vi "HEWH RLT PRAT.vi"() -> ()   [LabVIEW 2023] (continued)
            n1006 = call <vilib>:"Add State(s) to Queue__jki_lib_state_machine.vi"("State(s) in (\"\")"=w2472) -> ("States Out"=w2471:string)  [unwired: 14 in]
          }
          frame "Test: Update Display C" {
            n1007 = local read "Appliance Details C"() -> (w2473:T5)
            n1008 = local read "Current (C)"() -> (w2482:dbl)
            n1009 = Bundle By Name(cluster=w2483, "Station C Display.Display Data (RLT).Current Display"=w2482, "Station C Display.Appliance Details"=w2473) -> (w2481:T97)
            n1010 = Unbundle By Name(w2481) -> ("Station C Display.Display Data (RLT).Station Label Display"=w2479:string, "Station C Display.Display Data (RLT).Board ID Display"=w2478:string, "Station C Display.Display Data (RLT).Serial Number Display"=w2477:string, "Station C Display.Display Data (RLT).Current Display"=w2476:dbl, "Station C Display.Display Data (RLT).Status Color"=w2475:u32, "Station C Display.Display Data (RLT).Cycle Count Display"=w2474:i32)
            n1011 = property on="Station Label Display" class="Str"("Value"=w2479) -> ()  [unwired: 2 in, 2 out]
            n1012 = property on="Board ID Display" class="Str"("Value"=w2478) -> ()  [unwired: 2 in, 2 out]
            n1013 = property on="Serial Number Display" class="Str"("Value"=w2477) -> ()  [unwired: 2 in, 2 out]
            n1014 = property on="Current Display" class="DigNum (strict)"("Value"=w2476) -> ()  [unwired: 2 in, 2 out]
            n1015 = property on="Status Color" class="ColBox"("Value"=w2475) -> ()  [unwired: 2 in, 2 out]
            n1016 = property on="Cycle Count Display" class="DigNum (strict)"("Value"=w2474) -> ()  [unwired: 2 in, 2 out]
            n1017 = call <vilib>:"Add State(s) to Queue__jki_lib_state_machine.vi"("State(s) in (\"\")"=w2486) -> ("States Out"=w2485:string)  [unwired: 14 in]
          }
          frame "Test: Update Display D" {
            n1018 = local read "Appliance Details D"() -> (w2487:T5)
            n1019 = local read "Current (D)"() -> (w2496:dbl)
            n1020 = Bundle By Name(cluster=w2497, "Station D Display.Display Data (RLT).Current Display"=w2496, "Station D Display.Appliance Details"=w2487) -> (w2495:T97)
            n1021 = Unbundle By Name(w2495) -> ("Station D Display.Display Data (RLT).Station Label Display"=w2493:string, "Station D Display.Display Data (RLT).Board ID Display"=w2492:string, "Station D Display.Display Data (RLT).Serial Number Display"=w2491:string, "Station D Display.Display Data (RLT).Current Display"=w2490:dbl, "Station D Display.Display Data (RLT).Status Color"=w2489:u32, "Station D Display.Display Data (RLT).Cycle Count Display"=w2488:i32)
            n1022 = property on="Station Label Display" class="Str"("Value"=w2493) -> ()  [unwired: 2 in, 2 out]
            n1023 = property on="Board ID Display" class="Str"("Value"=w2492) -> ()  [unwired: 2 in, 2 out]
            n1024 = property on="Serial Number Display" class="Str"("Value"=w2491) -> ()  [unwired: 2 in, 2 out]
            n1025 = property on="Current Display" class="DigNum (strict)"("Value"=w2490) -> ()  [unwired: 2 in, 2 out]
            n1026 = property on="Status Color" class="ColBox"("Value"=w2489) -> ()  [unwired: 2 in, 2 out]
            n1027 = property on="Cycle Count Display" class="DigNum (strict)"("Value"=w2488) -> ()  [unwired: 2 in, 2 out]
            n1028 = call <vilib>:"Add State(s) to Queue__jki_lib_state_machine.vi"("State(s) in (\"\")"=w2500) -> ("States Out"=w2499:string)  [unwired: 14 in]
          }
          frame "Test: Wait for Power Off (Station A)" {
            # "I should use an event to change the condition value...its just more wires/\ncomplications...not sure its worth it."
            # "Need to add final conditions\nfor both 24hr and 1hr"
            n1029 = Unbundle By Name(w2540) -> ("Station A Display.Display Data (RLT)"=w2531:T32, "Draw Parameters Seq"=w2529:T48, "Current Cond A"=w2524:T2)  [unwired: 1 out]
            n1030 = local read item#-1() -> (w2505)
            n1031 = Unbundle By Name(w2505) -> ("TimerA (H:M:S)"=→"Timer 1", "TimerA (String)"=w2502, "Timer A"=w2501)
            "A Timer" <- w2501
            n1032 = local read "Core HEWH Data Input A"() -> (w2526:T13)
            n1033 = Bundle By Name(cluster=w2526, "Current Cond"=w2524) -> (w2525:T13)
            n1034 = local read "Draw Station"() -> (w2532:string)
            n1035 = local read "Start Draw"() -> (w2535:bool)
            n1036 = local read "Purge Time (Seconds)"() -> (w2506:dbl)
            n1037 = call "UTILITY String Notifier.vi"("Status"=UTILITY_Notifier."Set", "error in (no error)"=w2504, "Set Status"=w2502, "name (unnamed)"="TimerA") -> ("error out"=w2507:errorcluster)  [unwired: 6 in, 1 out]
            n1038 = call "HEWH Conditional Trigger.vi"("Draw Parameters Seq"=w2529, "Core HEWH Data Input"=w2525, "Station"="A", "Manual Draw Trigger"="Trigger Draw A", "Draw Station"=w2532, "Error In"=w2507, "Start Draw"=w2535, "Purge Time (sec)"=w2506, "Delay After Cutout (sec)"="Cutout Delay A (sec)", "A Timer"=w2501, "Disable Station in"="Disable Station 1", "StationA Setpoint"="StationA Setpoint", "Display Data (RLT) In"=w2531) -> ("Station Data Output"=w2510:T15, "Use Last Start Condition?"=→"Use Last Start Condition A?":bool, "SM States"=w2534:string, "Display Data (RLT) Out"=w2514:T32, "Core HEWH Data Output"=w2517:T13, "Disable Station"=w2521:bool, "Error Out"=w2527:errorcluster)  [unwired: 7 in, 1 out]
            n1039 = Unbundle By Name(w2517) -> ("Test Complete"=w2516:bool)
            "Test CompleteA" <- w2516
            n1040 = Unbundle By Name(w2517) -> ("Current Cond"=w2523:T2)
            "Condition A" <- w2523
            n1041 = call "HEWH End Of Test Display.vi"("String Notifier"="MessageA", "error in (no error)"=w2527, "Disable Station"=w2521, "Current Cond"=w2523) -> ("error out"=w2519:errorcluster, "Failure"=w2515:bool)  [unwired: 6 in]
            n1042 = Or(x=w2521, y=w2515) -> (x .or. y?=w2520:bool)
            n1043 = case shown="True" w2520 {
              tunnel: w2519 -> [w2550 w2555]
              tunnel: [w2550 w2554] -> w2518
              tunnel: w2516 -> [_ w2553]
              tunnel: w2515 -> [_ w2552]
              frame False {
              }
              frame True {
                n1044 = Or(x=w2553, y=w2552) -> (x .or. y?=w2551:bool)
                n1045 = case shown="True" w2551 {
                  tunnel: w2555 -> [w2557 w2560]
                  tunnel: [w2557 w2559] -> w2554
                  frame False {
                  }
                  frame True {
                    n1046 = flat-sequence {
                      tunnel: w2560 -> [w2563]
                      tunnel: [w2563] -> w2558
                      tunnel: [w2565] -> w2559
                      tunnel: w2558 -> [w2565]
                      frame #0 {
                        n1047 = local write "Log Data Output (A)"(FALSE ("Log Data Output (A)")) -> ()
                        n1048 = local write "Station ID to Reset"(Station_ID_Selector."A" ("Station ID to Reset")) -> ()
                      }
                      frame #1 {
                        "Final Headers A" <- TRUE ("Final Headers A")
                      }
                    }
                  }
                }
                n1049 = local write "Disable Station 1"(HEWH_RLT_Station_Disable."Disable Station (No Draw)" ("Disable Station 1")) -> ()
              }
            }
            n1050 = local read "Main Power"() -> (w2513:bool)
            n1051 = Bundle By Name(cluster=w2540, "Station A Display.Display Data (RLT)"=w2514, "Current Cond A"=w2523) -> (w2539:T97)
            n1052 = call "HEWH Check Power Set.vi"("Station Data Output"=w2510, "Timer"=w2501, "HEWH Power"=w2513) -> ("Set Power To This Value"=w2511:bool, "Trigger Power Set"=w2512:bool)  [unwired: 6 in, 1 out]
            n1053 = case shown="True" w2512 {
              tunnel: w2511 -> [_ w2547]
              frame False {
              }
              frame True {
                n1054 = property on="Main Power" class="Bool (strict)"("Val(Sgnl)"=w2547) -> ()  [unwired: 2 in, 2 out]
                n1055 = case shown="False" w2547 {
                  tunnel: ["Power OFF..." ("Set Status") "Power ON..." ("Set Status")] -> w2544
                  frame False {
                  }
                  frame True {
                  }
                }
                n1056 = call "UTILITY String Notifier.vi"("Status"=UTILITY_Notifier."Set", "Set Status"=w2544, "name (unnamed)"="MessageA") -> ()  [unwired: 7 in, 2 out]
              }
            }
            n1057 = call <vilib>:"Add State(s) to Queue__jki_lib_state_machine.vi"("State(s) in Front (\"\")"=w2534, "State(s) in (\"\")"=w2543) -> ("States Out"=w2542:string)  [unwired: 13 in]
          }
          frame "Test: Wait for Power Off (Station B)" {
            # "B Timer"
            # "Main Test Loop: Decides which Tank to Run, and starts that sequence."
            n1058 = Unbundle By Name(w2605) -> ("Station B Display.Display Data (RLT)"=w2595:T32, "Draw Parameters Seq"=w2602:T48, "Current Cond B"=w2589:T2)  [unwired: 1 out]
            n1059 = local read "Core HEWH Data Input B"() -> (w2591:T13)
            n1060 = local read item#-1() -> (w2569)
            n1061 = Unbundle By Name(w2569) -> ("TimerB (H:M:S)"=→"Timer 2", "TimerB (String)"=w2566, "Timer B"=w2568)
            "B Timer" <- w2568
            n1062 = Bundle By Name(cluster=w2591, "Current Cond"=w2589) -> (w2590:T13)
            n1063 = call "UTILITY String Notifier.vi"("Status"=UTILITY_Notifier."Set", "error in (no error)"=w2570, "Set Status"=w2566, "name (unnamed)"="TimerB") -> ("error out"=w2572:errorcluster)  [unwired: 6 in, 1 out]
            n1064 = local read "Purge Time (Seconds)"() -> (w2571:dbl)
            n1065 = local read "Draw Station"() -> (w2596:string)
            n1066 = local read "Start Draw"() -> (w2599:bool)
            n1067 = call "HEWH Conditional Trigger.vi"("Draw Parameters Seq"=w2602, "Core HEWH Data Input"=w2590, "Station"="B", "Manual Draw Trigger"="Trigger Draw B", "Draw Station"=w2596, "Error In"=w2572, "Start Draw"=w2599, "Purge Time (sec)"=w2571, "Delay After Cutout (sec)"="Cutout Delay B (sec)", "A Timer"=w2568, "Disable Station in"="Disable Station 2", "StationA Setpoint"="StationB Setpoint", "Display Data (RLT) In"=w2595) -> ("Station Data Output"=w2575:T15, "Use Last Start Condition?"=→"Use Last Start Condition B?":bool, "SM States"=w2598:string, "Display Data (RLT) Out"=w2594:T32, "Core HEWH Data Output"=w2581:T13, "Disable Station"=w2585:bool, "Error Out"=w2587:errorcluster)  [unwired: 7 in, 1 out]
            n1068 = Unbundle By Name(w2581) -> ("Test Complete"=w2580:bool)
            "Test CompleteB" <- w2580
            n1069 = Unbundle By Name(w2581) -> ("Current Cond"=w2588:T2)
            "Condition B" <- w2588
            n1070 = call "HEWH End Of Test Display.vi"("String Notifier"="MessageB" ("name (unnamed)"), "error in (no error)"=w2587, "Disable Station"=w2585, "Current Cond"=w2588) -> ("error out"=w2583:errorcluster, "Failure"=w2579:bool)  [unwired: 6 in]
            n1071 = Or(x=w2579, y=w2585) -> (x .or. y?=w2584:bool)
            n1072 = case shown="True" w2584 {
              tunnel: w2583 -> [w2615 w2620]
              tunnel: [w2615 w2619] -> w2582
              tunnel: w2580 -> [_ w2618]
              tunnel: w2579 -> [_ w2616]
              frame False {
              }
              frame True {
                n1073 = Or(x=w2618, y=w2616) -> (x .or. y?=w2617:bool)
                n1074 = case shown="True" w2617 {
                  tunnel: w2620 -> [w2622 w2625]
                  tunnel: [w2622 w2624] -> w2619
                  frame False {
                  }
                  frame True {
                    n1075 = flat-sequence {
                      tunnel: w2625 -> [w2628]
                      tunnel: [w2628] -> w2623
                      tunnel: [w2630] -> w2624
                      tunnel: w2623 -> [w2630]
                      frame #0 {
                        n1076 = local write "Log Data Output (B)"(FALSE ("Log Data Output (A)")) -> ()
                        n1077 = local write "Station ID to Reset"(Station_ID_Selector."B" ("Station ID to Reset")) -> ()
                      }
                      frame #1 {
                        "Final Headers B" <- TRUE ("Final Headers B")
                      }
                    }
                  }
                }
                n1078 = local write "Disable Station 2"(HEWH_RLT_Station_Disable."Disable Station (No Draw)" ("Disable Station 1")) -> ()
              }
            }
            n1079 = local read "Main Power"() -> (w2578:bool)
            n1080 = Bundle By Name(cluster=w2605, "Station B Display.Display Data (RLT)"=w2594, "Current Cond B"=w2588) -> (w2604:T97)
            n1081 = call "HEWH Check Power Set.vi"("Station Data Output"=w2575, "Timer"=w2568, "HEWH Power"=w2578) -> ("Set Power To This Value"=w2576:bool, "Trigger Power Set"=w2577:bool)  [unwired: 6 in, 1 out]
            n1082 = case shown="True" w2577 {
              tunnel: w2576 -> [_ w2609]
              frame False {
              }
              frame True {
                n1083 = property on="Main Power" class="Bool (strict)"("Val(Sgnl)"=w2609) -> ()  [unwired: 2 in, 2 out]
                n1084 = case shown="True" w2609 {
                  tunnel: ["Power OFF..." ("Set Status") "Power ON..." ("Set Status")] -> w2610
                  frame False {
                  }
                  frame True {
                  }
                }
                n1085 = call "UTILITY String Notifier.vi"("Status"=UTILITY_Notifier."Set", "Set Status"=w2610, "name (unnamed)"="MessageB") -> ()  [unwired: 7 in, 2 out]
              }
            }
            n1086 = call <vilib>:"Add State(s) to Queue__jki_lib_state_machine.vi"("State(s) in Front (\"\")"=w2598, "State(s) in (\"\")"=w2608) -> ("States Out"=w2607:string)  [unwired: 13 in]
          }
          frame "Test: Wait for Power Off (Station C)" {
            # "C Timer"
            # "Main Test Loop: Decides which Tank to Run, and starts that sequence."
            n1087 = local read "Core HEWH Data Input C"() -> (w2656:T13)
            n1088 = Unbundle By Name(w2670) -> ("Station C Display.Display Data (RLT)"=w2661:T32, "Draw Parameters Seq"=w2667:T48, "Current Cond C"=w2655:T2)  [unwired: 1 out]
            n1089 = local read item#-1() -> (w2634)
            n1090 = Unbundle By Name(w2634) -> ("TimerC (H:M:S)"=→"Timer 3", "TimerC (String)"=w2632, "Timer C"=w2631)
            "C Timer" <- w2631
            n1091 = Bundle By Name(cluster=w2656, "Current Cond"=w2655) -> (w2654:T13)
            n1092 = call "UTILITY String Notifier.vi"("Status"=UTILITY_Notifier."Set", "error in (no error)"=w2635, "Set Status"=w2632, "name (unnamed)"="TimerC") -> ("error out"=w2637:errorcluster)  [unwired: 6 in, 1 out]
            n1093 = local read "Purge Time (Seconds)"() -> (w2636:dbl)
            n1094 = local read "Draw Station"() -> (w2659:string)
            n1095 = local read "Start Draw"() -> (w2664:bool)
            n1096 = call "HEWH Conditional Trigger.vi"("Draw Parameters Seq"=w2667, "Core HEWH Data Input"=w2654, "Station"="C", "Manual Draw Trigger"="Trigger Draw C", "Draw Station"=w2659, "Error In"=w2637, "Start Draw"=w2664, "Purge Time (sec)"=w2636, "Delay After Cutout (sec)"="Cutout Delay C (sec)", "A Timer"=w2631, "Disable Station in"="Disable Station 3", "StationA Setpoint"="StationC Setpoint", "Display Data (RLT) In"=w2661) -> ("Station Data Output"=w2640:T15, "Use Last Start Condition?"=→"Use Last Start Condition C?":bool, "SM States"=w2663:string, "Display Data (RLT) Out"=w2660:T32, "Core HEWH Data Output"=w2646:T13, "Disable Station"=w2650:bool, "Error Out"=w2653:errorcluster)  [unwired: 7 in, 1 out]
            n1097 = Unbundle By Name(w2646) -> ("Current Cond"=w2651:T2)
            "Condition C" <- w2651
            n1098 = Unbundle By Name(w2646) -> ("Test Complete"=w2645:bool)
            "Test CompleteC" <- w2645
            n1099 = call "HEWH End Of Test Display.vi"("String Notifier"="MessageC" ("name (unnamed)"), "error in (no error)"=w2653, "Disable Station"=w2650, "Current Cond"=w2651) -> ("error out"=w2648:errorcluster, "Failure"=w2644:bool)  [unwired: 6 in]
            n1100 = local read "Main Power"() -> (w2643:bool)
            n1101 = Or(x=w2644, y=w2650) -> (x .or. y?=w2649:bool)
            n1102 = case shown="True" w2649 {
              tunnel: w2648 -> [w2680 w2685]
              tunnel: [w2680 w2684] -> w2647
              tunnel: w2645 -> [_ w2683]
              tunnel: w2644 -> [_ w2681]
              frame False {
              }
              frame True {
                n1103 = Or(x=w2683, y=w2681) -> (x .or. y?=w2682:bool)
                n1104 = case shown="True" w2682 {
                  tunnel: w2685 -> [w2687 w2690]
                  tunnel: [w2687 w2689] -> w2684
                  frame False {
                  }
                  frame True {
                    n1105 = flat-sequence {
                      tunnel: w2690 -> [w2693]
                      tunnel: [w2693] -> w2688
                      tunnel: [w2695] -> w2689
                      tunnel: w2688 -> [w2695]
                      frame #0 {
                        n1106 = local write "Log Data Output (C)"(FALSE ("Log Data Output (A)")) -> ()
                        n1107 = local write "Station ID to Reset"(Station_ID_Selector."C" ("Station ID to Reset")) -> ()
                      }
                      frame #1 {
                        "Final Headers C" <- TRUE ("Final Headers C")
                      }
                    }
                  }
                }
                n1108 = local write "Disable Station 3"(HEWH_RLT_Station_Disable."Disable Station (No Draw)" ("Disable Station 1")) -> ()
              }
            }
            n1109 = call "HEWH Check Power Set.vi"("Station Data Output"=w2640, "Timer"=w2631, "HEWH Power"=w2643) -> ("Set Power To This Value"=w2641:bool, "Trigger Power Set"=w2642:bool)  [unwired: 6 in, 1 out]
            n1110 = case shown="True" w2642 {
              tunnel: w2641 -> [_ w2674]
              frame False {
              }
              frame True {
                n1111 = property on="Main Power" class="Bool (strict)"("Val(Sgnl)"=w2674) -> ()  [unwired: 2 in, 2 out]
                n1112 = case shown="True" w2674 {
                  tunnel: ["Power OFF..." ("Set Status") "Power ON..." ("Set Status")] -> w2675
                  frame False {
                  }
                  frame True {
                  }
                }
                n1113 = call "UTILITY String Notifier.vi"("Status"=UTILITY_Notifier."Set", "Set Status"=w2675, "name (unnamed)"="MessageC") -> ()  [unwired: 7 in, 2 out]
              }
            }
            n1114 = Bundle By Name(cluster=w2670, "Station C Display.Display Data (RLT)"=w2660, "Current Cond C"=w2651) -> (w2669:T97)
            n1115 = call <vilib>:"Add State(s) to Queue__jki_lib_state_machine.vi"("State(s) in Front (\"\")"=w2663, "State(s) in (\"\")"=w2673) -> ("States Out"=w2672:string)  [unwired: 13 in]
          }
          frame "Test: Wait for Power Off (Station D)" {
            # "D Timer"
            # "Main Test Loop: Decides which Tank to Run, and starts that sequence."
            n1116 = Unbundle By Name(w2735) -> ("Station D Display.Display Data (RLT)"=w2725:T32, "Draw Parameters Seq"=w2732:T48, "Current Cond D"=w2719:T2)  [unwired: 1 out]
            n1117 = local read item#-1() -> (w2699)
            n1118 = Unbundle By Name(w2699) -> ("TimerD (H:M:S)"=→"Timer 4", "TimerD (String)"=w2698, "Timer D"=w2696)
            "D Timer" <- w2696
            n1119 = local read "Core HEWH Data Input D"() -> (w2721:T13)
            n1120 = local read "Purge Time (Seconds)"() -> (w2701:dbl)
            n1121 = Bundle By Name(cluster=w2721, "Current Cond"=w2719) -> (w2720:T13)
            n1122 = local read "Draw Station"() -> (w2724:string)
            n1123 = local read "Start Draw"() -> (w2729:bool)
            n1124 = call "UTILITY String Notifier.vi"("Status"=UTILITY_Notifier."Set", "error in (no error)"=w2700, "Set Status"=w2698, "name (unnamed)"="TimerD") -> ("error out"=w2702:errorcluster)  [unwired: 6 in, 1 out]
            n1125 = call "HEWH Conditional Trigger.vi"("Draw Parameters Seq"=w2732, "Core HEWH Data Input"=w2720, "Station"="D", "Manual Draw Trigger"="Trigger Draw D", "Draw Station"=w2724, "Error In"=w2702, "Start Draw"=w2729, "Purge Time (sec)"=w2701, "Delay After Cutout (sec)"="Cutout Delay D (sec)", "A Timer"=w2696, "Disable Station in"="Disable Station 4", "StationA Setpoint"="StationD Setpoint", "Display Data (RLT) In"=w2725) -> ("Station Data Output"=w2705:T15, "Use Last Start Condition?"=→"Use Last Start Condition D?":bool, "SM States"=w2728:string, "Display Data (RLT) Out"=w2726:T32, "Core HEWH Data Output"=w2711:T13, "Disable Station"=w2715:bool, "Error Out"=w2718:errorcluster)  [unwired: 7 in, 1 out]
            n1126 = Unbundle By Name(w2711) -> ("Current Cond"=w2716:T2)
            "Condition D" <- w2716
            n1127 = Unbundle By Name(w2711) -> ("Test Complete"=w2710:bool)
            "Test CompleteD" <- w2710
            n1128 = call "HEWH End Of Test Display.vi"("String Notifier"="MessageD" ("name (unnamed)"), "error in (no error)"=w2718, "Disable Station"=w2715, "Current Cond"=w2716) -> ("error out"=w2713:errorcluster, "Failure"=w2709:bool)  [unwired: 6 in]
            n1129 = Or(x=w2709, y=w2715) -> (x .or. y?=w2714:bool)
            n1130 = Bundle By Name(cluster=w2735, "Station D Display.Display Data (RLT)"=w2726, "Current Cond D"=w2716) -> (w2734:T97)
            n1131 = local read "Main Power"() -> (w2708:bool)
            n1132 = case shown="True" w2714 {
              tunnel: w2713 -> [w2745 w2750]
              tunnel: [w2745 w2749] -> w2712
              tunnel: w2710 -> [_ w2748]
              tunnel: w2709 -> [_ w2746]
              frame False {
              }
              frame True {
                n1133 = Or(x=w2748, y=w2746) -> (x .or. y?=w2747:bool)
                n1134 = case shown="True" w2747 {
                  tunnel: w2750 -> [w2752 w2755]
                  tunnel: [w2752 w2754] -> w2749
                  frame False {
                  }
                  frame True {
                    n1135 = flat-sequence {
                      tunnel: w2755 -> [w2758]
                      tunnel: [w2758] -> w2753
                      tunnel: [w2760] -> w2754
                      tunnel: w2753 -> [w2760]
                      frame #0 {
                        n1136 = local write "Log Data Output (D)"(FALSE ("Log Data Output (A)")) -> ()
                        n1137 = local write "Station ID to Reset"(Station_ID_Selector."D" ("Station ID to Reset")) -> ()
                      }
                      frame #1 {
                        "Final Headers D" <- TRUE ("Final Headers D")
                      }
                    }
                  }
                }
                n1138 = local write "Disable Station 4"(HEWH_RLT_Station_Disable."Disable Station (No Draw)" ("Disable Station 1")) -> ()
              }
            }
            n1139 = call "HEWH Check Power Set.vi"("Station Data Output"=w2705, "Timer"=w2696, "HEWH Power"=w2708) -> ("Set Power To This Value"=w2706:bool, "Trigger Power Set"=w2707:bool)  [unwired: 6 in, 1 out]
            n1140 = case shown="True" w2707 {
              tunnel: w2706 -> [_ w2739]
              frame False {
              }
              frame True {
                n1141 = property on="Main Power" class="Bool (strict)"("Val(Sgnl)"=w2739) -> ()  [unwired: 2 in, 2 out]
                n1142 = case shown="True" w2739 {
                  tunnel: ["Power OFF..." ("Set Status") "Power ON..." ("Set Status")] -> w2740
                  frame False {
                  }
                  frame True {
                  }
                }
                n1143 = call "UTILITY String Notifier.vi"("Status"=UTILITY_Notifier."Set", "Set Status"=w2740, "name (unnamed)"="MessageD") -> ()  [unwired: 7 in, 2 out]
              }
            }
            n1144 = call <vilib>:"Add State(s) to Queue__jki_lib_state_machine.vi"("State(s) in Front (\"\")"=w2728, "State(s) in (\"\")"=w2738) -> ("States Out"=w2737:string)  [unwired: 13 in]
          }
          frame "Check for UI Event" {
            n1145 = local read "Shutdown"() -> (w2765:string)
            n1146 = call <vilib>:"Add State(s) to Queue__jki_lib_state_machine.vi"("State(s) in Front (\"\")"=w2765, "State(s) in (\"\")"=w2766) -> ("States Out"=w2764:string)  [unwired: 13 in]
            n1147 = flat-sequence {
              tunnel: w2764 -> [w2769]
              tunnel: [w2769] -> w2763
              frame #0 {
                n1148 = local write "Shutdown"("" ("Shutdown")) -> ()
              }
            }
            n1149 = call <vilib>:"Add State(s) to Queue__jki_lib_state_machine.vi"("State(s) in (\"\")"=w2763) -> ("States Out"=w2768:string)  [unwired: 14 in]
          }
          frame "---------- Main Control ----------" {
            n1150 = call <vilib>:"Add State(s) to Queue__jki_lib_state_machine.vi"("State(s) in (\"\")"=w2772) -> ("States Out"=w2775:string)  [unwired: 14 in]
          }
          frame "Temp Decline A" {
            n1151 = Unbundle By Name(w2782) -> ("Draw Parameters Seq"=w2777:T48)
            n1152 = local read "Temp Decline Complete A"() -> (w2780:bool)
            n1153 = call "HEWH Temperature Decline.vi"("Error In"=w2778, "Station"="A", "Temp Decline Complete A"=w2780, "Draw Parameters Seq"=w2777) -> ("Error Out"=w2776:errorcluster, "Output States"=w2781:string)  [unwired: 5 in, 1 out]
            n1154 = call <vilib>:"Add State(s) to Queue__jki_lib_state_machine.vi"("State(s) in Front (\"\")"=w2781, "State(s) in (\"\")"=w2785) -> ("States Out"=w2784:string)  [unwired: 13 in]
          }
          frame "Temp Decline B" {
            n1155 = Unbundle By Name(w2792) -> ("Draw Parameters Seq"=w2791:T48)
            n1156 = local read "Temp Decline Complete B"() -> (w2787:bool)
            n1157 = call "HEWH Temperature Decline.vi"("Error In"=w2788, "Station"="B", "Temp Decline Complete A"=w2787, "Draw Parameters Seq"=w2791) -> ("Error Out"=w2786:errorcluster, "Output States"=w2790:string)  [unwired: 5 in, 1 out]
            n1158 = call <vilib>:"Add State(s) to Queue__jki_lib_state_machine.vi"("State(s) in Front (\"\")"=w2790, "State(s) in (\"\")"=w2795) -> ("States Out"=w2794:string)  [unwired: 13 in]
          }
          frame "Temp Decline C" {
            n1159 = Unbundle By Name(w2802) -> ("Draw Parameters Seq"=w2801:T48)
            n1160 = local read "Temp Decline Complete C"() -> (w2797:bool)
            n1161 = call "HEWH Temperature Decline.vi"("Error In"=w2798, "Station"="C", "Temp Decline Complete A"=w2797, "Draw Parameters Seq"=w2801) -> ("Error Out"=w2796:errorcluster, "Output States"=w2800:string)  [unwired: 5 in, 1 out]
            n1162 = call <vilib>:"Add State(s) to Queue__jki_lib_state_machine.vi"("State(s) in Front (\"\")"=w2800, "State(s) in (\"\")"=w2805) -> ("States Out"=w2804:string)  [unwired: 13 in]
          }
          frame "Temp Decline D" {
            n1163 = Unbundle By Name(w2812) -> ("Draw Parameters Seq"=w2811:T48)
            n1164 = local read "Temp Decline Complete D"() -> (w2807:bool)
            n1165 = call "HEWH Temperature Decline.vi"("Error In"=w2808, "Station"="D", "Temp Decline Complete A"=w2807, "Draw Parameters Seq"=w2811) -> ("Error Out"=w2806:errorcluster, "Output States"=w2810:string)  [unwired: 5 in, 1 out]
            n1166 = call <vilib>:"Add State(s) to Queue__jki_lib_state_machine.vi"("State(s) in Front (\"\")"=w2810, "State(s) in (\"\")"=w2815) -> ("States Out"=w2814:string)  [unwired: 13 in]
          }
          frame "Set Draw Station" {
            n1167 = Unbundle By Name(w2817) -> ("Draw Parameters Seq"=w2816:T48)
            n1168 = case shown="\"A\", Default" w2824 {
              selector: w2824 -> [w2836 _ _ _]
              tunnel: w2823 -> [w2841 w2846 w2851 w2856]
              tunnel: [w2840 w2845 w2850 w2855] -> w2825
              tunnel: w2821 -> [w2839 _ _ _]
              tunnel: w2820 -> [_ w2844 _ _]
              tunnel: w2819 -> [_ _ w2848 _]
              tunnel: w2818 -> [_ _ _ w2852]
              tunnel: w2816 -> [w2837 w2842 w2849 w2854]
              frame "A", Default {
                n1169 = local read "GEA2_A?"() -> (w2838:bool)
                n1170 = call "HEWH Draw Start GEA3 Commands.vi"("Draw Station"=w2836, "GEA3?"=w2838, "error in (no error)"=w2841, "Draw Parameters Seq"=w2837, "GEA3 Reference Out"=w2839) -> ("error out"=w2840:errorcluster)  [unwired: 5 in, 1 out]
              }
              frame "B" {
                n1171 = local read "GEA2_B?"() -> (w2843:bool)
                n1172 = call "HEWH Draw Start GEA3 Commands.vi"("GEA3?"=w2843, "error in (no error)"=w2846, "Draw Parameters Seq"=w2842, "GEA3 Reference Out"=w2844) -> ("error out"=w2845:errorcluster)  [unwired: 6 in, 1 out]
              }
              frame "C" {
                n1173 = local read "GEA2_C?"() -> (w2847:bool)
                n1174 = call "HEWH Draw Start GEA3 Commands.vi"("GEA3?"=w2847, "error in (no error)"=w2851, "Draw Parameters Seq"=w2849, "GEA3 Reference Out"=w2848) -> ("error out"=w2850:errorcluster)  [unwired: 6 in, 1 out]
              }
              frame "D" {
                n1175 = local read "GEA2_D?"() -> (w2853:bool)
                n1176 = call "HEWH Draw Start GEA3 Commands.vi"("GEA3?"=w2853, "error in (no error)"=w2856, "Draw Parameters Seq"=w2854, "GEA3 Reference Out"=w2852) -> ("error out"=w2855:errorcluster)  [unwired: 6 in, 1 out]
              }
            }
            n1177 = for {
              N: 10 -> [_]
              tunnel: w2824 -> [w2831]
              shift-right: [w2833] -> w2826
              shift-left: w2825 -> [w2832]
              n1178 = Wait Until Next ms Multiple(millisecond multiple=u32 100) -> ()  [unwired: 1 out]
              n1179 = call "UTILITY String Notifier.vi"("Status"=UTILITY_Notifier."Set", "error in (no error)"=w2832, "Set Status"=w2831, "name (unnamed)"="Draw Station") -> ("error out"=w2833:errorcluster)  [unwired: 6 in, 1 out]
            }
            n1180 = call <vilib>:"Add State(s) to Queue__jki_lib_state_machine.vi"("State(s) in (\"\")"=w2829) -> ("States Out"=w2828:string)  [unwired: 14 in]
            "Draw Station" <- w2824
          }
          frame "-------Dispense Algorithm--------" {
            n1181 = call <vilib>:"Add State(s) to Queue__jki_lib_state_machine.vi"("State(s) in (\"\")"=w2861) -> ("States Out"=w2860:string)  [unwired: 14 in]
          }
          frame "Dispense Gallons" {
            n1182 = Unbundle By Name(w2892) -> ("Current Cond A"=w2867:T2, "Current Cond B"=w2866:T2, "Current Cond C"=w2865:T2, "Current Cond D"=w2864:T2, "Draw Parameters Seq.Station A.Flow Rate (GPM)"=→"GPM Target (Station A)":dbl, "Draw Parameters Seq.Station B.Flow Rate (GPM)"=→"GPM Target (Station B)":dbl, "Draw Parameters Seq.Station C.Flow Rate (GPM)"=→"GPM Target (Station C)":dbl, "Draw Parameters Seq.Station D.Flow Rate (GPM)"=→"GPM Target (Station D)":dbl, "Draw Parameters Seq.Station A.Temperature (F)"=→"Degree Setting( Station A)":dbl, "Draw Parameters Seq.Station B.Temperature (F)"=→"Degree Setting( Station B)":dbl, "Draw Parameters Seq.Station C.Temperature (F)"=→"Degree Setting( Station C)":dbl, "Draw Parameters Seq.Station D.Temperature (F)"=→"Degree Setting( Station D)":dbl, "Draw Parameters Seq.Station D.Condition Value #1"=w2877:dbl, "Draw Parameters Seq.Station C.Condition Value #1"=w2878:dbl, "Draw Parameters Seq.Station B.Condition Value #1"=w2879:dbl, "Draw Parameters Seq.Station A.Condition Value #1"=w2880:dbl, "Draw Parameters Seq.Station A.Terminate Condition"=w2876:T17, "Draw Parameters Seq.Station B.Terminate Condition"=w2875:T17, "Draw Parameters Seq.Station C.Terminate Condition"=w2874:T17, "Draw Parameters Seq.Station D.Terminate Condition"=w2872:T17, "Draw Parameters Seq"=w2873:T48)
            n1183 = call "HEWH Update Draw Amount Display.vi"("Terminate Condition A"=w2876, "Terminate Condition B"=w2875, "Terminate Condition C"=w2874, "Terminate Condition D"=w2872, "Error In"=w2882, "Gallons to Draw A"=w2880, "Gallons to Draw B"=w2879, "Gallons to Draw C"=w2878, "Gallons to Draw D"=w2877) -> ("Draw Amount (Station A)"=→"Draw Amount (Station A)":dbl, "Draw Amount (Station B)"=→"Draw Amount (Station B)":dbl, "Draw Amount (Station C)"=→"Draw Amount (Station C)":dbl, "Draw Amount (Station D)"=→"Draw Amount (Station D)":dbl, "Error Out"=w2881:errorcluster)  [unwired: 6 in]
            n1184 = flat-sequence {
              tunnel: [w2911] -> w2898
              tunnel: w2881 -> [w2910]
              tunnel: [w2910] -> w2897
              tunnel: w2895 -> [w2909]
              tunnel: [w2909] -> w2894
              tunnel: w2873 -> [w2908]
              tunnel: [w2907] -> w2891
              tunnel: w2867 -> [w2906]
              tunnel: w2866 -> [w2905]
              tunnel: w2865 -> [w2904]
              tunnel: w2864 -> [w2903]
              tunnel: [w2902] -> w2863
              tunnel: [w2901] -> w2862
              tunnel: w2898 -> [w2948]
              tunnel: [w2952] -> w2896
              tunnel: w2897 -> [w2954]
              tunnel: w2894 -> [w2955]
              tunnel: [w2953] -> w2893
              tunnel: w2891 -> [w2947]
              tunnel: w2863 -> [w2946]
              tunnel: w2862 -> [w2945]
              frame #0 {
                n1185 = local read "Draw Station"() -> (w2912:string)
                n1186 = case shown="\"D\"" w2912 {
                  tunnel: [Station_ID_Selector."A" ("Station ID") Station_ID_Selector."B" ("Station ID") Station_ID_Selector."C" ("Station ID") Station_ID_Selector."D" ("Station ID")] -> w2911
                  tunnel: w2908 -> [w2919 w2927 w2935 w2941]
                  tunnel: [w2917 w2926 w2934 w2944] -> w2907
                  tunnel: w2906 -> [w2914 _ _ _]
                  tunnel: w2905 -> [_ w2922 _ _]
                  tunnel: w2904 -> [_ _ w2930 _]
                  tunnel: w2903 -> [_ _ _ w2938]
                  tunnel: [w2914 w2922 w2930 w2938] -> w2902
                  tunnel: [w2913 w2921 w2929 w2937] -> w2901
                  frame "A", Default {
                    n1187 = Unbundle By Name(w2919) -> ("Station A"=w2918:T15)
                    n1188 = local read "Disable Purge Pressurization A"() -> (w2913:bool)
                    n1189 = local read "Station A Test Sequence"() -> (w2915:T15[])
                    n1190 = local read "Use Last Start Condition A?"() -> (w2916:bool)
                    n1191 = call "HEWH Set Draw Station.vi"("Use Last Start Condition?"=w2916, "Station"=w2918, "Station Test Sequence"=w2915) -> ("Station Set"=w2917:T15)  [unwired: 7 in, 1 out]
                  }
                  frame "B" {
                    n1192 = Unbundle By Name(w2927) -> ("Station B"=w2924:T15)
                    n1193 = local read "Use Last Start Condition B?"() -> (w2923:bool)
                    n1194 = local read "Disable Purge Pressurization B"() -> (w2921:bool)
                    n1195 = local read "Station B Test Sequence"() -> (w2925:T15[])
                    n1196 = call "HEWH Set Draw Station.vi"("Use Last Start Condition?"=w2923, "Station"=w2924, "Station Test Sequence"=w2925) -> ("Station Set"=w2926:T15)  [unwired: 7 in, 1 out]
                  }
                  frame "C" {
                    n1197 = Unbundle By Name(w2935) -> ("Station C"=w2932:T15)
                    n1198 = local read "Disable Purge Pressurization C"() -> (w2929:bool)
                    n1199 = local read "Station C Test Sequence"() -> (w2933:T15[])
                    n1200 = local read "Use Last Start Condition C?"() -> (w2931:bool)
                    n1201 = call "HEWH Set Draw Station.vi"("Use Last Start Condition?"=w2931, "Station"=w2932, "Station Test Sequence"=w2933) -> ("Station Set"=w2934:T15)  [unwired: 7 in, 1 out]
                  }
                  frame "D" {
                    n1202 = Unbundle By Name(w2941) -> ("Station D"=w2940:T15)
                    n1203 = local read "Station D Test Sequence"() -> (w2942:T15[])
                    n1204 = local read "Use Last Start Condition D?"() -> (w2939:bool)
                    n1205 = local read "Disable Purge Pressurization D"() -> (w2937:bool)
                    n1206 = call "HEWH Set Draw Station.vi"("Use Last Start Condition?"=w2939, "Station"=w2940, "Station Test Sequence"=w2942) -> ("Station Set"=w2944:T15)  [unwired: 7 in, 1 out]
                  }
                }
              }
              frame #1 {
                n1207 = Bundle By Name(cluster=T81 {"Start Draw"=FALSE, "Station ID"=enum."A", "Station Draw Info"={"Sequence #"=0.0, "Cycles"=0, "Mode Setting"="", "Flow Rate (GPM)"=0.0, "Temperature (F)"=0.0, "Reset Timer"=FALSE, "Use Temp Decline Method"=FALSE, "Terminate Condition"=enum."C1-Terminate Draw @ Gallon Mark", "Condition Value #1"=0.0, "UE"=FALSE, "LE"=FALSE, "Comp"=FALSE, "Fan"=FALSE, "Test End Time (Sec)"=0.0, "Purge Until Cutout"=FALSE, "Start Conditions"=enum."Heat Source Cutout", "Condition Value #2"=0.0, "Remove Power"=FALSE, "Time"=0.0, "Check Special Cond."=enum."SC2-Check Heat Source (On-C2/Off-C1)", "Condition#"=enum."C1", "Draw Flags"=enum."N/A", "Data Processing Delay (FHD 15sec, UEF 5 Sec)"=0.0, "Test Complete"=FALSE, "User Setpoint"=0.0, "Tank Setpoint"=0.0}, "Send Condition"=enum."N/A", "Disable Purge Pressurization"=FALSE}, "Send Condition"=w2946, "Start Draw"=TRUE, "Station ID"=w2948, "Station Draw Info"=w2947, "Disable Purge Pressurization"=w2945) -> (w2949:T81)
                n1208 = Enqueue Element(queue=w2955, element=w2949, error in (no error)=w2954) -> (queue out=w2953:refnum<queue>, error out=w2952:errorcluster)  [unwired: 1 in, 1 out]
                "Station Draw Info" <- w2947
              }
            }
            n1209 = call <vilib>:"Add State(s) to Queue__jki_lib_state_machine.vi"("State(s) in (\"\")"=w2900) -> ("States Out"=w2899:string)  [unwired: 14 in]
          }
        }
        n1210 = case shown="False" "Debug" {
          tunnel: [w1864 w1867] -> w1854
          tunnel: w1853 -> [w1864 w1866]
          tunnel: w1851 -> [_ w1865]
          frame False {
          }
          frame True {
            n1211 = Build Array (concatenate)(w1866, w1865) -> (w1867:string[])
          }
        }
        "Main Control" <- w1854
        "MainLoop" <- w1846
      }
      "Finish" <- w1835
      n1212 = property on="Finish" class="Bool (strict)"("Val(Sgnl)"=w1835) -> ()  [unwired: 2 in, 2 out]
      n1213 = Release Queue(queue=w1833, error in (no error)=w1832) -> (error out=→"Error Out":errorcluster)  [unwired: 1 in, 2 out]
    }
    frame Enabled {
    }
  }
  n1214 = call "Create User Event - Stop.vi"("error in (no error)"=w74) -> ("error out"=w60:errorcluster, "User Event - Stop"=w68:refnum<user-event>)  [unwired: 9 in]
  n1215 = register-events(w68) -> (reference out=w67:refnum<event-registration>, error out=w70:errorcluster)  [unwired: 2 in]
  n1216 = call "Create All Message Queues.vi"("error in (no error)"=w60) -> ("error out"=w31:errorcluster, "Message Queues out"=w32:T101)  [unwired: 9 in]
  n1217 = disable-structure shown="Disabled" {
    disable-tunnel: w96 -> [w2964 _]
    disable-tunnel: w93 -> [w2963 _]
    disable-tunnel: w92 -> [w2962 _]
    disable-tunnel: w91 -> [w2961 _]
    disable-tunnel: w90 -> [w2960 _]
    disable-tunnel: w89 -> [w2959 _]
    disable-tunnel: w88 -> [w2958 _]
    disable-tunnel: w82 -> [w2957 _]
    disable-tunnel: w57 -> [w2956 _]
    frame Disabled {
      # "Handle User Events (button clicks, ect)"
      n1218 = call <vilib>:"Add State(s) to Queue__jki_lib_state_machine.vi"("State(s) in (\"\")"="Data: Initialize") -> ("States Out"=w2966:string)  [unwired: 14 in]
      n1219 = while "UI Events" {
        shift-right: [w2977] -> _
        shift-left: _ -> [w2976]
        shift-right: [w2980] -> _
        shift-left: w2956 -> [w2975]
        shift-right: [w2979] -> _
        shift-left: w2966 -> [w2981]
        tunnel: w2964 -> [w2974]
        tunnel: w2959 -> [w2973]
        tunnel: w2958 -> [w2972]
        tunnel: w2963 -> [w2971]
        tunnel: w2962 -> [w2970]
        tunnel: w2961 -> [w2969]
        tunnel: w2960 -> [w2968]
        tunnel: w2957 -> [w2967]
        stop <- w2978 stop-if-true
        # "UI Events"
        n1220 = call <vilib>:"Parse State Queue__JKI_lib_State_Machine.vi"("State Queue"=w2981, "Error In (no error)"=w2975) -> ("Remaining States"=w2983:string, "Current State"=w2984:string, "Arguments"=w2982:string)  [unwired: 11 in]
        "UI State" <- w2984
        n1221 = case shown="\"Error Handler\"" w2984 {
          selector: w2984 -> [_ _ w3283 _ _ _ _ _ _ _ _ _ _]
          tunnel: w2983 -> [w2998 w3282 w3287 w3299 w3304 w3308 w3325 w3342 w3347 w3355 w3382 w3385 w3405]
          tunnel: w2982 -> [_ _ _ _ _ _ _ _ _ _ _ _ _]
          tunnel: w2976 -> [w2996 w3279 w3285 w3296 w3302 w3305 _ w3339 w3344 w3350 w3379 w3383 w3401]
          tunnel: [w2995 w3280 w3289 errorcluster {"status"=FALSE, "code"=0, "source"=""} ("error out") w3301 w3306 w3314 w3340 w3345 w3351 w3380 w3384 w3403] -> w2980
          tunnel: w2975 -> [w2994 w3280 w3288 w3295 w3301 w3306 w3311 w3340 w3345 w3352 w3380 w3384 w3389]
          tunnel: [w2997 w3281 w3286 w3298 w3303 w3307 w3324 w3341 w3346 w3354 w3381 w3385 w3405] -> w2979
          tunnel: [_ _ _ _ TRUE _ _ _ _ _ _ _ _] -> w2978
          tunnel: [w2993 w3279 w3285 w3296 w3302 w3305 w3318 w3339 w3344 w3348 w3379 w3383 w3404] -> w2977
          tunnel: w2974 -> [w2990 _ _ _ _ _ _ _ _ w3349 _ _ _]
          tunnel: w2973 -> [w2992 _ _ _ _ _ _ _ _ _ _ _ _]
          tunnel: w2972 -> [w2991 _ _ _ _ _ _ _ _ _ _ _ _]
          tunnel: w2971 -> [w2989 _ _ _ _ _ _ _ _ _ _ _ _]
          tunnel: w2970 -> [w2988 _ _ _ _ _ _ _ _ _ _ _ _]
          tunnel: w2969 -> [w2987 _ _ _ _ _ _ _ _ _ _ _ _]
          tunnel: w2968 -> [w2986 _ _ _ _ _ _ _ _ _ _ _ _]
          tunnel: w2967 -> [_ _ _ _ _ _ w3309 _ _ _ _ _ _]
          frame "", "Idle" {
            w2985 = 250  # Timeout
            n1222 = event shown="[2] \"Station A Display.Display Data (RLT).UI Button\": Value Change" {
              selector: _ -> [_ _ _ _ _ _ _ _]
              dyn-events: _ -> [_ _ _ _ _ _ _ _]
              timeout: w2985 -> [_ _ _ _ _ _ _ _]
              tunnel: w2998 -> [w3005 w3029 w3064 w3123 w3180 w3237 w3267 w3270]
              tunnel: [w3004 w3030 w3064 w3123 w3180 w3237 w3266 w3269] -> w2997
              tunnel: w2996 -> [w3000 w3031 w3065 w3124 w3181 w3238 w3264 w3272]
              tunnel: [w3003 w3027 w3058 w3116 w3174 w3231 w3265 w3274] -> w2995
              tunnel: w2994 -> [w3003 w3027 w3062 w3122 w3179 w3236 w3265 w3274]
              tunnel: [w2999 w3031 w3065 w3124 w3181 w3238 w3264 w3271] -> w2993
              tunnel: w2992 -> [_ _ w3057 w3115 w3173 w3229 _ _]
              tunnel: w2991 -> [_ _ w3052 w3111 w3168 w3225 _ _]
              tunnel: w2990 -> [_ _ _ _ _ _ _ _]
              tunnel: w2989 -> [_ _ w3041 _ _ _ _ _]
              tunnel: w2988 -> [_ _ _ w3098 _ _ _ _]
              tunnel: w2987 -> [_ _ _ _ w3156 _ _ _]
              tunnel: w2986 -> [_ _ _ _ _ w3213 _ _]
              event Timeout {
                n1223 = event-data() -> ()  [unwired: 1 in, 1 out]
                n1224 = case shown="True" "AUTO STEP" {
                  tunnel: [w3007 w3020] -> w3002
                  tunnel: w3000 -> [w3008 w3013]
                  tunnel: [w3008 w3012] -> w2999
                  frame False {
                    n1225 = local read "Start ANSI UI"() -> (w3006:bool)
                    n1226 = case shown="True" w3006 {
                      tunnel: ["" ("State(s) in Front (\"\")") "Get Rates" ("State(s) in Front (\"\")")] -> w3007
                      frame False {
                      }
                      frame True {
                      }
                    }
                  }
                  frame True {
                    n1227 = local read "Proportioning\nValve"() -> (w3011:dbl)
                    n1228 = call "UTILITY E-Time.vi"() -> ("Elapsed Time (sec)"=w3017:dbl)  [unwired: 9 in, 2 out]
                    n1229 = Round Toward -Infinity(1:w3017) -> (0:w3016:dbl)
                    n1230 = Quotient & Remainder(x=w3016, y="Proportioning Valve Step Time (Sec)") -> (x-y*floor(x/y)=w3019:dbl)  [unwired: 1 out]
                    n1231 = To Word Integer(number=w3019) -> (16bit integer=w3018:i16)
                    n1232 = Equal To 0?(x=w3018) -> (x = 0?=w3015:bool)
                    n1233 = case shown="True" w3015 {
                      tunnel: ["" ("State(s) in Front (\"\")") "Mix Valve Step Control" ("State(s) in Front (\"\")")] -> w3020
                      tunnel: w3013 -> [w3021 w3025]
                      tunnel: [w3021 w3024] -> w3012
                      tunnel: w3011 -> [_ w3023]
                      frame False {
                      }
                      frame True {
                        n1234 = Bundle By Name(cluster=w3025, "User Controls.Proportional Valve"=w3023) -> (w3024:T103)
                      }
                    }
                  }
                }
                n1235 = call <vilib>:"Add State(s) to Queue__jki_lib_state_machine.vi"("State(s) in Front (\"\")"=w3002, "State(s) in (\"\")"=w3005) -> ("States Out"=w3004:string)  [unwired: 13 in]
              }
              event "Finish": Value Change {
                n1236 = event-data() -> ()  [unwired: 1 in, 6 out]
                n1237 = call <vilib>:"Add State(s) to Queue__jki_lib_state_machine.vi"("State(s) in Front (\"\")"="Exit" ("State(s) in Front (\"\")"), "State(s) in (\"\")"=w3029) -> ("States Out"=w3030:string)  [unwired: 13 in]
              }
              event Value Change {
                # "This is a pop-up screen to allow the\nuser to log data and save a test"
                n1238 = event-data() -> ()  [unwired: 1 in, 6 out]
                n1239 = local read "Core HEWH Data Input A"() -> (w3051:T13)
                n1240 = Unbundle By Name(w3041) -> ("Display Data (RLT).Station Label Display"=w3040:string)
                n1241 = local read "Station A Test Sequence"() -> (w3053:T15[])
                n1242 = local read "Scan Rate (Seconds)"() -> (w3035:T11)
                n1243 = property on="Start/Pause test" class="Bool (strict)"("DisabledEnum"=T87."Enabled" ("Disabled")) -> ()  [unwired: 2 in, 2 out]
                n1244 = Bundle By Name(cluster=T89 {"Test Fixture Hardware"={"Power "={"Yokogawa"={"WT210"={"Sample Rate (1: 0.25s)"=0, "A Range (12: 20A)"=0, "V Range (6: 600V)"=0, "Power VISA Yokogawa WT210"=""}, "WT500"={"Power VISA Yokogawa WT500"="", "V Range (8: 1000V)"=0, "I Range (7: 40A)"=0, "Update Rate (3: 500ms)"=0}, "WT310_2"={"Sample Rate (1: 0.25s)"=0, "A Range (12: 20A)"=0, "V Range (6: 600V)"=0, "Power VISA Yokogawa WT310_2"=""}, "WT310_3"={"Sample Rate (1: 0.25s)"=0, "A Range (12: 20A)"=0, "V Range (6: 600V)"=0, "Power VISA Yokogawa WT310_3"=""}}, "Aplus"={"Aplus IP Address"="", "Remote Port"=0, "Instrument"="", "Instr Driver Revision"=""}, "Power Limits"={"Crest Factor"={"Upper Limit"=0.0, "Lower Limit"=0.0}, "Harmonic Content"={"Uthd"=0.0}, "Voltage"={"% Error"=0.0}, "Stability"={"<1 Watt "={"Wattage"=0.0, "Slope (mW/H)"=0.0}, ">1 Watt"={"1%Power/Hour"=0.0}}}, "Nominal Voltage"=0, "Time Limit (s)"=0.0, "Power Variation Limit (%)"=0.0, "Power Supply"={"Chroma 61605"="", "Use Chroma?"=FALSE}}, "Weight Scale"={"Com Options"={"IND560Scale VISA"="", "IP Address"="", "Remote Port"=0, "Setra Scale VISA"="", "GSE 350"=""}, "Select Scale"=""}, "Flow Rates"={"Laurel Cold IP Address"="", "Laurel Hot IP Address"="", "Hot Water Laurel VISA"="", "Cold Water Laurel VISA"="", "Remote Port"=0, "Laurel Communication Type"="", "Meters To Collect (Hot Cold)"="", "HOT Laurel Reference"=refnum, "COLD Laurel Reference"=refnum, "Modbus Hot Ref"=refnum}, "Analog Data"={"Agilent"={"Agilent 34972_1"="", "Agilent 34972_2"="", "Agilent 34972_3"="", "Agilent 34972_4"="", "Agilent 34972_5"="", "Agilent 34972_6"="", "Agilent Gain"=0.0, "TC Type (K,J,T)"="", "Instrument IDN?"="", "TC Channels-List"="", "Analog Channels-List"="", "Agilent Cluster Array"=[], "TC Channels-List 2"="", "Analog Channels-List 2"=""}, "Yokogawa"={"MW100"="", "Intellifaucet"=FALSE}, "Select Analog"="", "TC Coefficients"={"TC Coefficients 1"=[], "TC Coefficients 2"=[], "TC Coefficients 3"=[], "TC Coefficients 4"=[], "TC Coefficients 5"=[], "TC Coefficients 6"=[], "TC Coefficients 7"=[]}, "NI Tasks (Dryer DOE)"=[], "Laurel Analog"={"Laurel IP (Water Temp)"="", "Laurel IP (Pressure)"=""}}, "Viasala Temperature & Humidity"={"IP Address 1"="", "Remote Port"=0, "IP Address 2"="", "IP Address 3"="", "Viasala Modbus"=refnum, "Probe Number"=0}, "Gas Meter"={"Gas Meter 1"="", "Gas Meter 2"="", "Gas Meter 3"="", "Gas Meter 4"="", "Gas Meter 5"="", "Gas Meter 6"="", "Data Frame Format"={"Absolute Pressure"=FALSE, "Gauge/Diff. Pressure"=FALSE, "Barometric Pressure"=FALSE, "Temperature"=FALSE, "Volumetric"=FALSE, "Mass"=FALSE, "Setpoint"=FALSE, "Valve Drive"=FALSE, "Totalizer"=FALSE, "Totalizer Timer"=FALSE, "Totalizer Average Flow"=FALSE, "Totalizer Peak Flow"=FALSE, "Gas Selected"=FALSE, "Tot. Timer Format"=0}, "Measurement Units"={"Software Rev"="", "Model Number"="", "Manufacturer Info"="", "Software Sub-Rev"="", "Board Rev"="", "Units of Measure Input"={"Abs. Pressure"="", "Gauge/Diff. Press."="", "Barometric Press."="", "Temperature"="", "Volume"="", "Mass"="", "Setpoint"="", "Valve Drive"="", "Totalizer"="", "Tot. Timer"="", "Tot. Avg. Flow"="", "Tot. Peak Flow"=""}}, "Ritter Gas Meter 1"=""}, "Barometric Pressure"={"HEISE 901A"="", "Use Barometer?"=FALSE}, "Gas Analysis"={"Ultramat 23 VISA"=""}, "Inficon Micro GC"={"Propane IP Address"="192.168.1.33", "Natural Gas  IP Address"="192.168.1.32", "Remote Port"=502, "Natural Modbus"=refnum, "Propane Modbus"=refnum}, "Tenney Environmental Chamber"={"Remote Port"=0, "IP Address"="", "Tenney Modbus"=refnum}}, "GEA2"={"Address"=0, "Source"=0, "Viper/Hawk"=0}, "DOE Capacity Measurments"={"Weight 1"=0.0, "Model Number 1"="", "Temp 1"=0.0, "Serial Number 1"="", "Lab Number 1"="", "Lab Number 2"="", "Serial Number 2"="", "Temp 2"=0.0, "Model Number 2"="", "Weight 2"=0.0, "Lab Number 3"="", "Serial Number 3"="", "Temp 3"=0.0, "Model Number 3"="", "Weight 3"=0.0, "Lab Number 4"="", "Serial Number 4"="", "Temp 4"=0.0, "Model Number 4"="", "Weight 4"=0.0, "Capacity Measurment Output String"=[]}, "Initialize.Washer In"={"Appliance Details"={"FileVersionInfo"={"FileVersion"="", "ProductName"="", "InternalName"="", "CompanyName"="", "LegalCopyright"="", "FileDescription"=""}, "Dishwasher Info"={"Open Cup Weight (gm):"=0.0, "Auto Cup Weight (gm):"=0.0, "Detergent-Dish:"="", "Inlet Temperature-Dish:"="", "Cycle Mode-Dish:"="", "Unit Control-Dish:"="", "Manufacturer-Dish:"=""}, "Washer Info"={"Hot Water Temperature (Fahrenheit):"="", "Cold Water Temperature (Fahrenheit):"="", "Capacity (cu.ft):"=0.0, "Initial Cloth Weight:"=0.0, "Cloth Lot:"=0, "Model Family:"="", "Program Name:"="", "Cycle Selection:"="", "Wash Temperature:"="", "Rinse Temperature:"="", "Load Size:"=""}, "File Name Output Array"=[], "Calibration Output Array"=[], "Appliance Common"={"Engineer:"="", "Model Number:"="", "Serial Number:"="", "Comments:"="", "Station ID:"="", "Technician:"="", "TR Number:"="", "Lab ID:"="", "Voltage:"="", "Water Pressure (PSI):"="", "Test Date:"="", "Computer Name:"="", "IP Address:"="", "Ambient RH:"="", "Frequency:"="", "Build:"="", "Filename:"="", "Test Type:"="", "Load Run #:"=0, "Ambient Temperature (F):"="", "File Path:"=path "", "Cycles Per Year"=0}, "Water Heater"={"Heating Mode:"=""}, "Dryer"={"Heat Setting:"="", "Washer Water Temperature (60 ± 5°F):"=0, "Water Hardness (PPM):"=0, "Dryness Setting:"="", "Dryer Type:"="", "Exhaust:"="", "Drying Cycle:"="", "Load Type:"="", "Nominal Load Weight"="", "Dryer Initial IMC Data"={"Measured IMC (lbs)"=0.0, "Actual Initial RMC (%)"=0.0, "RMC (Desired %)"=0.0, "Bone Dry Wt(lbs)"=0.0, "Tolerance(%)"=0.0, "Actual Final RMC (%)"=0.0, "CEF (lbf/kWh)"=0.0, "Minimum Weight (lbf)"=0.0, "Average Weight (lbf)"=0.0, "Maximum Weight (lbf)"=0.0, "Measured IMC In Range?"=FALSE, "Moisture Reduction Factor"=0.0, "Field Use Factor"=0.0, "Empty Dryer Cold Weigth"=0.0, "Energy Standard"=enum."D2-Automatic Dryer", "Weight Cloth (lbs)"=0.0, "Relative Moisture Content (%)"=0.0, "Relative Moisture Content - Avg (%)"=0.0}}}, "Display Data (RLT)"={"Status Color"=0, "Serial Number Display"="", "Cycle Count Display"=0, "Station Label Display"="", "Current Run Start Time Display"=0.0, "Board ID Display"="", "RPM Display"=0, "Current Display"=0.0, "Current Path Display"=path "", "Saving Display"=FALSE, "Unit Type Display"=enum."", "Total Time On Display"=0.0, "UI Button"=FALSE}}} ("Washer Controls In"), "Initialize.Washer In.Display Data (RLT).Station Label Display"=w3040) -> (w3042:T89)
                n1245 = Unbundle By Name(w3051) -> ("LV Program"=w3038:T25)
                n1246 = case shown="\"HEWH\", \"Gas Water Heater\"" w3038 {
                  tunnel: ["A" ("Station Input") w3067] -> w3061
                  frame Default {
                  }
                  frame "HEWH", "Gas Water Heater" {
                    n1247 = local read "Station"() -> (w3067:string)
                  }
                }
                n1248 = local read "File Locations A"() -> (w3050:T3)
                n1249 = call "PRAT Test Setup.vi"("Station Input"=w3061, "Test Sequence Input"=w3053, "Input Scan Rate"=w3035, "Washer Controls In"=w3042, "Filepath In"=w3050, "Error In"=w3062, "LV Program"=w3038) -> ("Cutout Delay (sec)"=w3046:dbl, "NOx Purge Time Out"=w3032:dbl, "Disable Purge Pressurization Output"=w3037:bool, "Unit Setpoint Out"=w3044:i32, "Appliance Details"=w3048:T5, "Filepath Out"=w3049:T3, "Station ID"=w3060:T26, "Log Data Output"=w3047:bool, "Temperature Decline Amount (°F)"=w3034:dbl, "Final Output"=w3063:T15[], "PRAT Test.ctlCancel Output"=w3056:bool, "Scan Rate Output"=w3036:dbl, "Test Procedure"=w3039:string, "Reset Cycle Count"=w3055:bool, "New Cycle Count Out"=w3054:i32, "Purge Time (s)"=w3033:dbl, "Error Out"=w3059:errorcluster)  [unwired: 4 in]
                n1250 = local write "Updated Cycle Count"(w3054) -> ()
                n1251 = local write "Reset Cycle Count"(w3055) -> ()
                n1252 = case shown="False" w3056 {
                  tunnel: w3063 -> [w3088 _]
                  tunnel: w3060 -> [w3087 _]
                  tunnel: w3059 -> [w3084 w3090]
                  tunnel: [w3075 w3090] -> w3058
                  tunnel: w3057 -> [w3085 _]
                  tunnel: w3052 -> [w3081 _]
                  tunnel: w3049 -> [w3076 _]
                  tunnel: w3048 -> [w3080 _]
                  tunnel: w3047 -> [w3077 _]
                  tunnel: w3046 -> [w3079 _]
                  tunnel: w3044 -> [w3074 _]
                  tunnel: w3039 -> [w3073 _]
                  tunnel: w3037 -> [w3069 _]
                  tunnel: w3036 -> [w3068 _]
                  tunnel: w3034 -> [w3072 _]
                  tunnel: w3033 -> [w3071 _]
                  tunnel: w3032 -> [w3070 _]
                  frame False {
                    n1253 = local write "Station ID to Reset"(w3087) -> ()
                    n1254 = local write "StationA Setpoint"(w3074) -> ()
                    n1255 = local write "Cutout Delay A (sec)"(w3079) -> ()
                    n1256 = local write "NOx Purge Time"(w3070) -> ()
                    n1257 = local write "Temperature Decline Amount (°F)"(w3072) -> ()
                    n1258 = local write "Purge Time (Seconds)"(w3071) -> ()
                    n1259 = local write "Disable Station 1"(HEWH_RLT_Station_Disable."Enable Station" ("Disable Station 1")) -> ()
                    n1260 = case shown="True" w3069 {
                      frame False {
                      }
                      frame True {
                        n1261 = local write "Pressurization Time (sec)"(0 ("Pressurization Time (sec)")) -> ()
                      }
                    }
                    n1262 = property on="Scan Rate (Seconds)" class="DigNum (strict)"("Value"=w3068) -> ()  [unwired: 2 in, 2 out]
                    n1263 = Generate User Event(user event=w3085, event data cluster=TRUE ("event data"), error in=w3084) -> (error out=w3082:errorcluster)  [unwired: 1 in, 1 out]
                    n1264 = Generate User Event(user event=w3081, event data cluster=TRUE ("event data"), error in=w3082) -> (error out=w3075:errorcluster)  [unwired: 1 in, 1 out]
                    "Station A Test Sequence" <- w3088
                    "Appliance Details A" <- w3080
                    "Updated File Path A" <- w3076
                    "Log Data Output (A)" <- w3077
                    "Test Procedure" <- w3073
                    "Disable Purge Pressurization A" <- w3069
                  }
                  frame True {
                  }
                }
              }
              event Value Change {
                n1265 = event-data() -> ()  [unwired: 1 in, 6 out]
                n1266 = Unbundle By Name(w3098) -> ("Display Data (RLT).Station Label Display"=w3100:string)
                n1267 = local read "Core HEWH Data Input B"() -> (w3110:T13)
